vi "acceptDisableCommand.vi"(8 "error in (no error)":errorcluster, 11 "SALCommunicator in":refnum<class "SALCommunicatorDL.lvclass">) -> (0 "error out":errorcluster, 2 "Command ID":i32, 3 "SALCommunicator out":refnum<class "SALCommunicatorDL.lvclass">)   [LabVIEW 2016, in "SALCommunicatorDL.lvclass"]
uses:
  SALCommunicatorDL.lvclass
  ts_sallv_exa/SALLV_EXA.lvlib
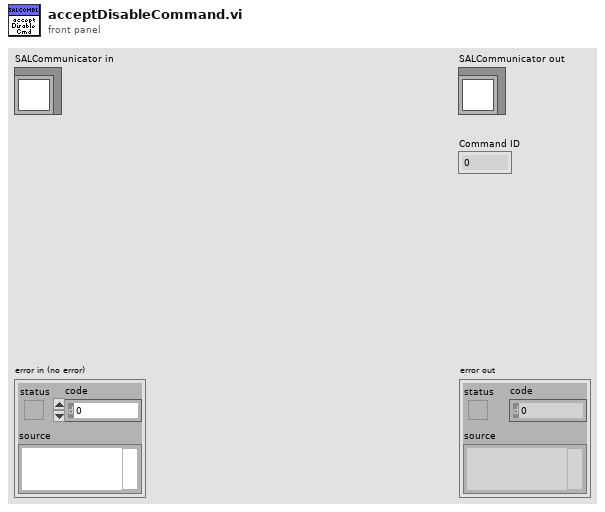
[diagram p1: front panel]
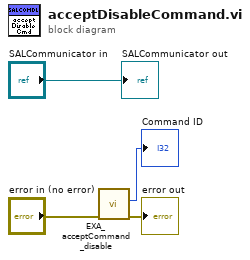
[diagram p0: block diagram]
diagram:
  n1 = call "EXA_acceptCommand_disable.vi"("error in (no error)"="error in (no error)") -> ("error out"=→"error out":errorcluster, "function return"=→"Command ID":i32)  [unwired: 8 in, 1 out]
  "SALCommunicator out" <- "SALCommunicator in"
